vi "closeFPGAVIRef.vi"(8 "error in (no error)":errorcluster, 11 "ComponentData in":refnum<class "ComponentData.lvclass">) -> (0 "error out":errorcluster, 3 "ComponentData out":refnum<class "ComponentData.lvclass">)   [LabVIEW 2013, in "ComponentData.lvlib" / "ComponentData.lvclass"]
uses:
  <userlib>/Common/Component/Application/RT/ComponentData/ComponentData/ComponentData.lvclass
  <vilib>/FPGAPlugInAG/cRIO-9074/niLvFpga_Close_cRIO-9074.vi
  <vilib>/rvi/interface/nirviCloseFPGA/nirviCloseFPGA.xnode
  <userlib>/Common/Component/Application/RT/ComponentData/ComponentData/fpgaVIRefCRIO9074.ctl
  <userlib>/Common/Component/Application/RT/ComponentData.lvlib
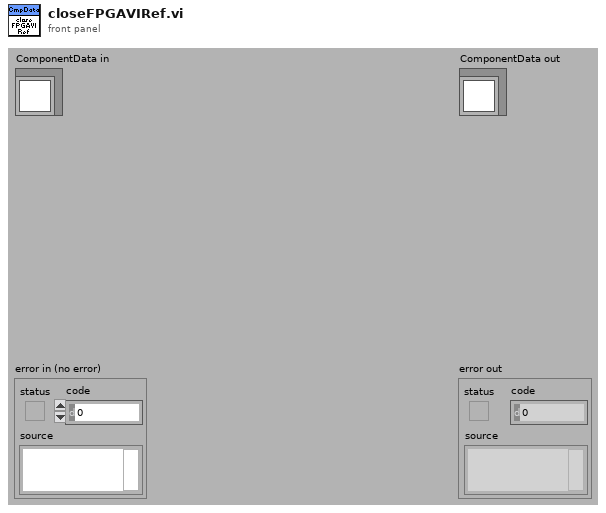
[diagram p1: front panel]
types:
  T1 = typedef "ComponentData.lvlib/fpgaVIRefCRIO9074.ctl" = refnum<k20>
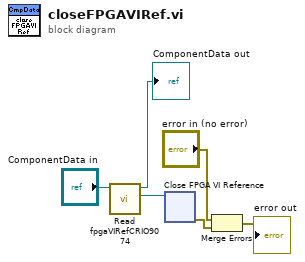
[diagram p0: block diagram]
diagram:
  n1 = call <userlib>:"Read fpgaVIRefCRIO9074.vi"("ComponentData in"="ComponentData in") -> ("fpgaVIRefCRIO9074"=w4:T1, "ComponentData out"=→"ComponentData out":refnum<class "ComponentData.lvclass">)  [unwired: 8 in, 1 out]
  n2 = xnode "Close FPGA VI Reference"("FPGA VI Reference In"=w4) -> ("error out"=w2:errorcluster)  [unwired: 1 in]
  n3 = Merge Errors("error in (no error)", w2) -> (→"error out":errorcluster)
